vi "Save Blocks - PM.vi"   [LabVIEW 2014]
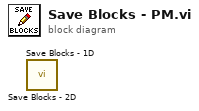
[diagram p0: block diagram]
diagram:
  n1 = call "Save Blocks - 2D.vi"() -> ()  [unwired: 10 in, 2 out]
  n2 = call "Save Blocks - 1D.vi"() -> ()  [unwired: 10 in, 2 out]
